vi "RAD2DEG.vi"(9 "IN (DEG)":dbl, 10 "IN (RAD)":dbl) -> (1 "OUT (RAD)":dbl, 2 "OUT (DEG)":dbl)   [LabVIEW 2014, in "Manipulator.lvclass"]
uses:
  Manipulator.lvclass
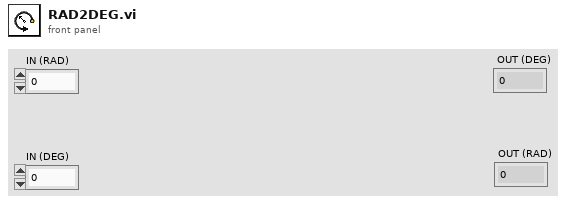
[diagram p1: front panel]
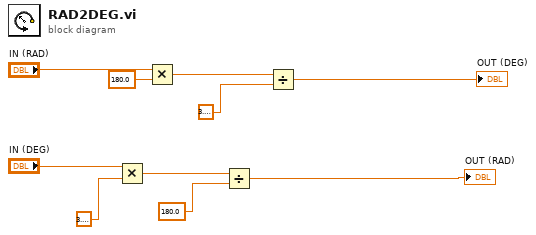
[diagram p0: block diagram]
diagram:
  n1 = Multiply(x="IN (DEG)", y=3.141592653589793) -> (x*y=w3:dbl)
  n2 = Multiply(x="IN (RAD)", y=180.0) -> (x*y=w8:dbl)
  n3 = Divide(x=w3, y=180.0) -> (x/y=→"OUT (RAD)":dbl)
  n4 = Divide(x=w8, y=3.141592653589793) -> (x/y=→"OUT (DEG)":dbl)
